vi "LSCI 370 Action Scan.vi"(0 "VISA session":refnum<visa-resource-name>, 5 "Scan Channel (1)":i32=1 min=1 max=16 step=1, 7 "Autoscan (F: Autoscan Off)":bool, 11 "error in (no error)":errorcluster) -> (4 "dup VISA session":refnum<visa-resource-name>, 15 "error out":errorcluster)   [LabVIEW 2016]
doc: "This VI selects which channel to switch the scanner to and configures the autoscan feature. Functions only when the Model 3716 Scanner is installed."
panel:
  # "Autoscan On\nAutoscan Off"
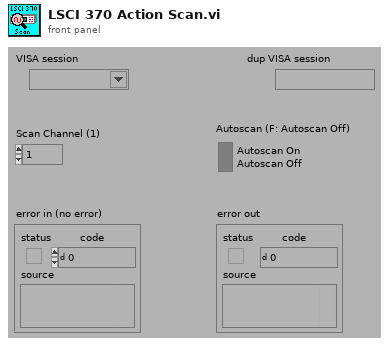
[diagram p1: front panel]
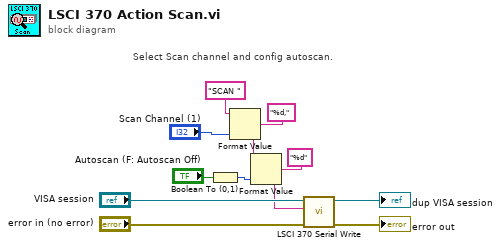
[diagram p0: block diagram]
diagram:
  # "Select Scan channel and config autoscan."
  n1 = Boolean To (0,1)(Boolean="Autoscan (F: Autoscan Off)") -> (0, 1=w2:i16)
  n2 = Format Value(string ("")="SCAN ", format string="%d,", value (0)="Scan Channel (1)") -> (output string=w4:string)
  n3 = Format Value(string ("")=w4, format string="%d", value (0)=w2) -> (output string=w1:string)
  n4 = call "LSCI 370 Serial Write.vi"("error in (no error)"="error in (no error)", "Write Buffer (\"\")"=w1, "VISA session"="VISA session") -> ("error out"=→"error out":errorcluster, "dup VISA session"=→"dup VISA session":refnum<visa-resource-name>)  [unwired: 6 in, 1 out]
